vi "pierwsze zadanie.vi"() -> ()   [LabVIEW 2020]
panel:
  in  "Jaka liczba":dbl=60.0 format="%#_13g"
  out "Ilosc wylosowan":i32
  out "output array":dbl[](array[numeric])
  out "Aktualnie wylosowana":dbl
  # "Aktualnie wylosowana"
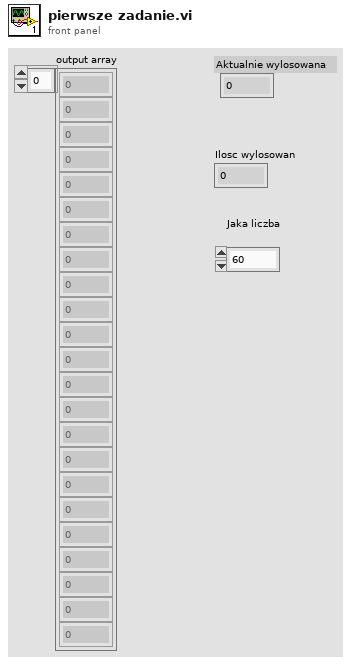
[diagram p1: front panel]
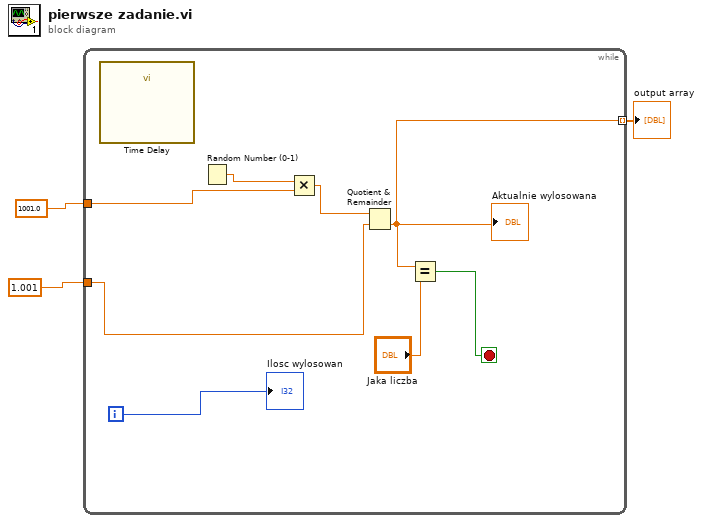
[diagram p0: block diagram]
diagram:
  n1 = while {
    tunnel: 1001.0 -> [w10]
    tunnel: 1.001 -> [w9]
    tunnel: [w4] -> w1 mode=indexing
    i -> [w5]
    stop <- w7 stop-if-true
    n2 = call "Time Delay"() -> ()  [unwired: 11 in, 1 out]
    n3 = Random Number (0-1)() -> (number: 0 to 1=w6:dbl)
    n4 = Multiply(x=w6, y=w10) -> (x*y=w11:dbl)
    n5 = Quotient & Remainder(x=w11, y=w9) -> (floor(x/y)=w4:dbl)  [unwired: 1 out]
    "Aktualnie wylosowana" <- w4
    n6 = Equal?(x=w4, y="Jaka liczba") -> (x = y?=w7:bool)
    "Ilosc wylosowan" <- w5
  }
  "output array" <- w1
